vi "Get Data Type Name.vi"(11 "IAttribute Data Type View in":refnum<class "IAttribute Data Type View.lvclass">) -> (3 "Data Type Name":string="Default Data Type")   [LabVIEW 2017, in "IAttribute Data Type View.lvclass"]
uses:
  <vilib>/gpm_packages/@cs/Test-executive-builder/Source/Test Executive Builder Dialogs/IAttribute Data Type View/IAttribute Data Type View.lvclass
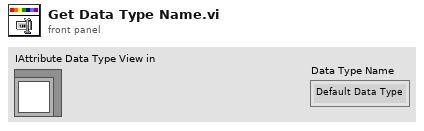
[diagram p1: front panel]
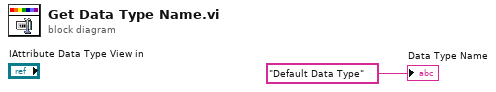
[diagram p0: block diagram]
diagram:
  "Data Type Name" <- "Default Data Type"
